vi "move puzzle.vi"(4 "upper white row":i32, 5 "solve":picture[][](array[picture]), 7 "current state":picture[][](array[picture]), 8 "currentselected peice column":i32, 9 "current selected peice row":i32, 10 "lower white coordinate":i32, 11 "allow peice movement":bool) -> (2 "puzzle finished":bool, 3 "updated image array":picture[][](array[picture]))   [LabVIEW 2014]
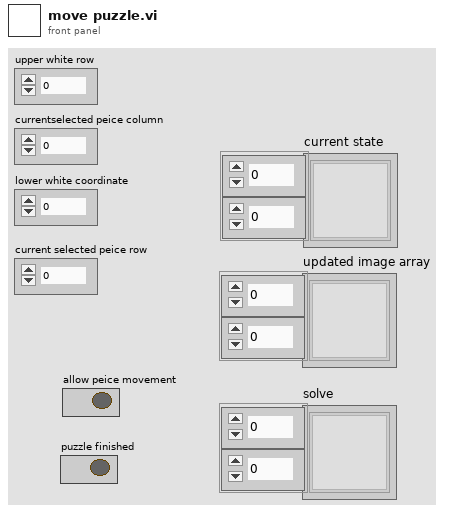
[diagram p1: front panel]
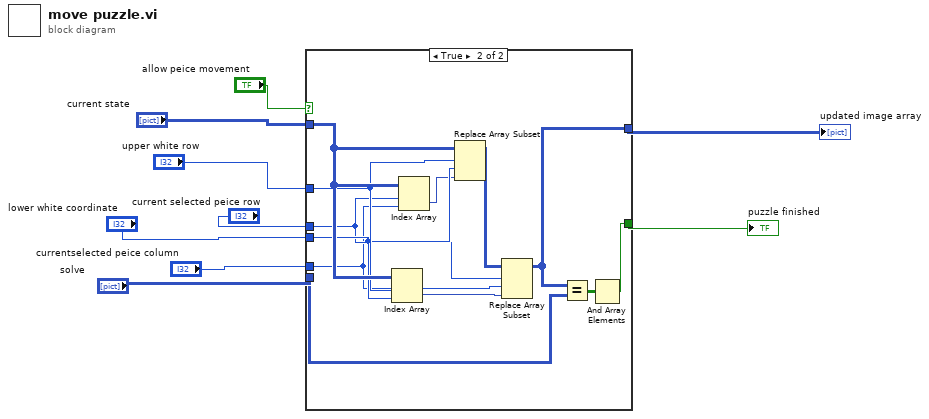
[diagram p0: block diagram]
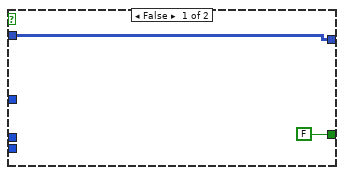
[diagram p2: hidden frame]
diagram:
  n1 = case shown="True" "allow peice movement" {
    tunnel: "current state" -> [w11 w23]
    tunnel: "upper white row" -> [_ w22]
    tunnel: "lower white coordinate" -> [_ w21]
    tunnel: "current selected peice row" -> [_ w18]
    tunnel: "currentselected peice column" -> [_ w17]
    tunnel: [w11 w12] -> w7
    tunnel: "solve" -> [_ w13]
    tunnel: [FALSE w14] -> w9
    frame False {
    }
    frame True {
      n2 = Index Array(array=w23, index (row)=w22, index (col)=w21) -> (element=w16:picture)
      n3 = Index Array(array=w23, index (row)=w18, index (col)=w17) -> (element=w20:picture)
      n4 = Replace Array Subset(array=w23, new element=w20, index (row)=w22, index (col)=w21) -> (w19:picture[][])
      n5 = Replace Array Subset(array=w19, new element=w16, index (row)=w18, index (col)=w17) -> (w12:picture[][])
      n6 = Equal?(x=w12, y=w13) -> (x = y?=w15:bool[][])
      n7 = And Array Elements(Boolean array=w15) -> (logical AND=w14:bool)
    }
  }
  "puzzle finished" <- w9
  "updated image array" <- w7
